vi "DAQ-Sync and Start.vi"(9 "Manage skip samples?":bool=TRUE, 11 "error in (no error)":errorcluster) -> (15 "error out":errorcluster)   [LabVIEW 2020]
uses:
  AODO/Typedefs/AODO-Action.ctl
  AIDI/Typedefs/AIDI-Action.ctl
  Counter/Typedefs/CTR-Action.ctl
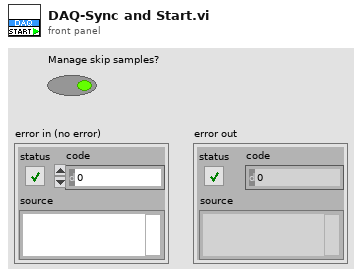
[diagram p1: front panel]
types:
  T1 = typedef "CTR-Action.ctl" = enum16{"Clear", "Configure", "Initialize", "Init & Start", "Start", "Clean up"}
  T2 = typedef "AODO-Action.ctl" = enum16{"Configure", "Initialize", "Start", "Write", "Clean up", "Init & Start", "Config & Test", "Position", "Set AO Gains", "Zero", "Prime", "Status"}
  T3 = typedef "AIDI-Action.ctl" = enum16{"Configure", "Initialize", "Start", "Read", "Clean up", "Init & Start", "Config & Test", "Position", "Skip"}
  T4 = typedef "AODO-Config.ctl" = cluster{"AO":T5, "DO":T6, "hold outputs":bool, "ExtTrig":bool, "Trig Src":string, "regen":bool, "finite":bool}
  T5 = typedef "AODO-Output Spec.ctl" = cluster{"Channels":string[], "Fs (Hz)":dbl, "Npts":i32, "Gains":dbl[]}
  T6 = typedef "DO-Output Spec.ctl" = cluster{"Channels":string[], "Fs (Hz)":dbl, "Npts":i32, "Port":string}
  T7 = typedef "AODO-Task Specification.ctl" = cluster{"Task":refnum<k21>, "Channels":string, "Dual channel":bool, "Index":i32[]}
  T8 = typedef "AIDI-Config.ctl" = cluster{"AI":T9, "DI":T10, "ExtTrig":bool}
  T9 = typedef "AIDI-Output Spec.ctl" = cluster{"Channels":string[], "Fs (Hz)":dbl, "Npts":i32}
  T10 = typedef "DI-Output Spec.ctl" = cluster{"Channels":string[], "Fs (Hz)":dbl, "Npts":i32, "Port":string}
  T11 = typedef "AIDI-Task Specification.ctl" = cluster{"Task":refnum<k21>, "Channels":string, "Dual channel":bool, "Index":i32[]}
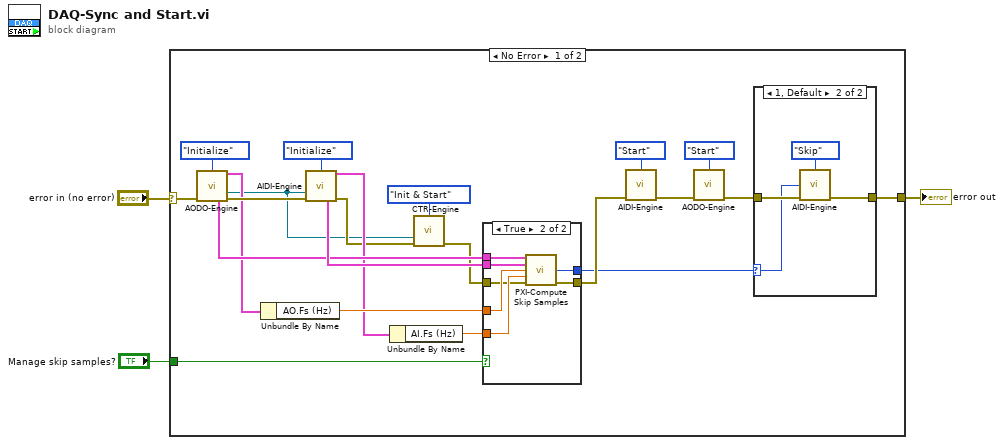
[diagram p0: block diagram]
diagram:
  n1 = case shown="No Error" "error in (no error)" {
    selector: "error in (no error)" -> [w24 w39]
    tunnel: [w8 w39] -> w2
    tunnel: "Manage skip samples?" -> [w18 _]
    frame No Error {
      n2 = call "AODO-Engine.vi"("Action"=AODO-Action."Initialize", "error in (no error)"=w24) -> ("Config out"=w15:T4, "Sync Task"=w4:refnum<k21>, "Tasks Out"=w16:T7[], "error out"=w23:errorcluster)  [unwired: 9 in, 1 out]
      n3 = Unbundle By Name(w15) -> ("AO.Fs (Hz)"=w14:dbl)
      n4 = call "AIDI-Engine.vi"("Action"=AIDI-Action."Initialize", "Sync task in"=w4, "error in (no error)"=w23) -> ("Config Out"=w13:T8, "Tasks Out"=w17:T11[], "error out"=w6:errorcluster)  [unwired: 7 in, 3 out]
      n5 = Unbundle By Name(w13) -> ("AI.Fs (Hz)"=w12:dbl)
      n6 = call "CTR-Engine.vi"("action"=CTR-Action."Init & Start", "Sync task in"=w4, "error in (no error)"=w6) -> ("error out"=w5:errorcluster)  [unwired: 12 in]
      n7 = case shown="True" w18 {
        tunnel: w16 -> [_ w38]
        tunnel: w17 -> [_ w37]
        tunnel: w14 -> [_ w36]
        tunnel: w12 -> [_ w35]
        tunnel: w5 -> [w31 w34]
        tunnel: [w31 w33] -> w11
        tunnel: [_ w32] -> w10
        frame False {
        }
        frame True {
          n8 = call "PXI-Compute Skip Samples.vi"("AO Tasks"=w38, "AI Tasks"=w37, "AO Sample Rate"=w36, "AI Sample Rate"=w35, "error in (no error)"=w34) -> ("Skip Samples"=w32:i32, "error out"=w33:errorcluster)  [unwired: 9 in]
        }
      }
      n9 = call "AIDI-Engine.vi"("Action"=AIDI-Action."Start", "error in (no error)"=w11) -> ("error out"=w20:errorcluster)  [unwired: 8 in, 5 out]
      n10 = call "AODO-Engine.vi"("Action"=AODO-Action."Start", "error in (no error)"=w20) -> ("error out"=w9:errorcluster)  [unwired: 9 in, 4 out]
      n11 = case shown="1, Default" w10 {
        selector: w10 -> [_ w27]
        tunnel: w9 -> [w26 w29]
        tunnel: [w26 w28] -> w8
        frame 0 {
        }
        frame 1, Default {
          n12 = call "AIDI-Engine.vi"("Action"=AIDI-Action."Skip", "Nskip"=w27, "error in (no error)"=w29) -> ("error out"=w28:errorcluster)  [unwired: 7 in, 5 out]
        }
      }
    }
    frame Error {
    }
  }
  "error out" <- w2
